vi "ConnectionNextNumber.vi"(10 "Reset":bool) -> (2 "ConnectionNextNumber":u32)   [LabVIEW 2022 SP3, in "Connection.lvlib" / "Connection.lvclass"]
uses:
  Connection.lvclass
  Connection.lvclass/Connection.ctl
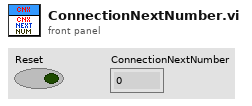
[diagram p1: front panel]
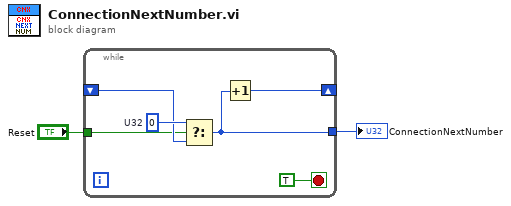
[diagram p0: block diagram]
diagram:
  n1 = while {
    shift-right: [w7] -> _
    shift-left: _ -> [w5]
    tunnel: "Reset" -> [w4]
    tunnel: [w3] -> w1
    stop <- TRUE stop-if-true
    w6 = u32 0  # U32
    n2 = Select(t=w6, s=w4, f=w5) -> (s? t:f=w3:u32)
    n3 = Increment(x=w3) -> (x+1=w7:u32)
  }
  "ConnectionNextNumber" <- w1
